vi "Test Periodic.vi"() -> ()   [LabVIEW 2016]
uses:
  SubSystems/Drive/Drive System.lvlib
  Vision/Vision Drive/Vision Drive.lvlib
  SubSystems/Path Track/Path Track.lvlib
panel:
  in  "Setting":enum16{"Custom", "Boiler", "Gear"}(ring)
  in  "Custom":i32
  in  "Offset":dbl format="%#_13g"
  in  "y":dbl=1.0
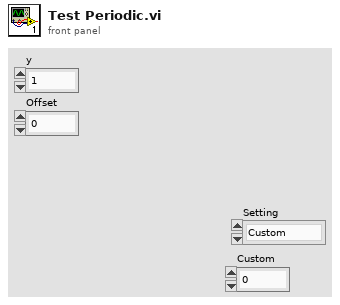
[diagram p1: front panel]
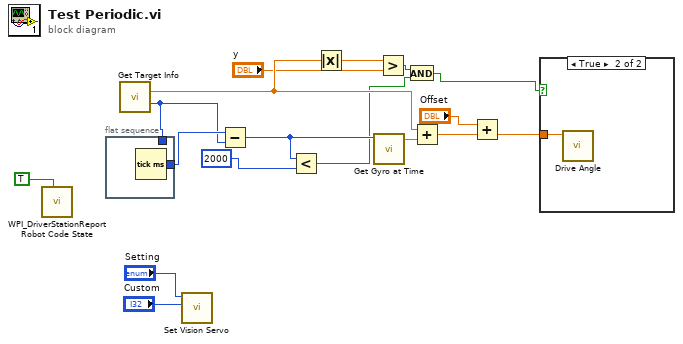
[diagram p0: block diagram]
diagram:
  n1 = call <vilib>:"WPI_DriverStationReport Robot Code State.vi"("Test"=TRUE ("Autonomous")) -> ()  [unwired: 10 in, 1 out]
  n2 = flat-sequence {
    tunnel: [w18] -> w16
    tunnel: w13 -> [_]
    frame #0 {
      n3 = Tick Count (ms)() -> (millisecond timer value=w18:u32)
    }
  }
  n4 = call "Get Target Info.vi"() -> ("Angle (deg)"=w12:dbl, "timestamp"=w13:u32)  [unwired: 11 in, 3 out]
  n5 = call "Set Vision Servo.vi"("Custom"="Custom", "Setting"="Setting") -> ()  [unwired: 9 in, 1 out]
  n6 = Subtract(x=w16, y=w13) -> (x-y=w9:u32)
  n7 = Less?(x=w9, y=u32 2000) -> (x < y?=w7:bool)
  n8 = Absolute Value(x=w12) -> (abs(x)=w5:dbl)
  n9 = call "Get Gyro at Time.vi"("Get ms ago"=w9) -> ("Angle"=w17:dbl)  [unwired: 9 in, 1 out]
  n10 = Greater?(x=w5, y="y") -> (0:w8:bool)
  n11 = And(x=w8, y=w7) -> (x .and. y?=w6:bool)
  n12 = Add(x=w12, y=w17) -> (x+y=w15:dbl)
  n13 = Add(x="Offset", y=w15) -> (x+y=w4:dbl)
  n14 = case shown="True" w6 {
    tunnel: w4 -> [_ w19]
    frame False {
    }
    frame True {
      n15 = call "Drive Angle.vi"("Angle"=w19) -> ()  [unwired: 10 in, 1 out]
    }
  }
